vi "OpenSourceRIO.vi"() -> ()   [LabVIEW 2019]
uses:
  Controls/AnalogTrigger_Sources.ctl
  Controls/AnalogTrigger_Limits.ctl
  Controls/Encoder_Configs.ctl
  Controls/Encoder_Config.ctl
  Helpers/Source.ctl
  Controls/Encoder_TimerConfigs.ctl
  Controls/TimerConfig.ctl
  Controls/Interrupt_Configs.ctl
  Controls/DutyCycle_Sources.ctl
  Controls/Counter_TimerConfigs.ctl
  Controls/Counter_Configs.ctl
  Controls/Counter_Config.ctl
  Controls/Encoder_Output.ctl
  Helpers/TimerOutput.ctl
  Controls/Counter_Output.ctl
  Helpers/AnalogTriggerOutput.ctl
  <vilib>/Platform/TimedLoop/XDataNode/timing_clust.ctl
  <vilib>/Platform/TimedLoop/XDataNode/nitl_modes.ctl
  <vilib>/Platform/TimedLoop/XDataNode/wakeup.ctl
  <vilib>/rvi/Emulation/niFpgaGetClockAttributes.vi
  <vilib>/rvi/Emulation/niFpgaSctlEmulationGetInTimedLoop.vi
  <vilib>/rvi/Emulation/niFpgaEmulationReportErrorSimple.vi
  <vilib>/rvi/Emulation/niFpgaCriticalErrorInLSC.vi
  <vilib>/rvi/eio/common/nirviEmuTemplateMethod_errors.vi
  <vilib>/rvi/Emulation/niFpgaProcessEmulError.vi
  <vilib>/rvi/eio/common/nirviEmuTemplatePropertyGet_noerrors.vi
  <vilib>/rvi/occurrence/nirviWaitOnOccurrenceBase.vi
  <vilib>/eio/EIONode/EIONode.xnode
  <vilib>/eio/EIOPropertyNode/EIOPropertyNode.xnode
  <vilib>/platform/TimedLoop/XDataNode/XDataNode.xnode
  <vilib>/Platform/TimedLoop/XDataNode/XDNodeRunTimeDep.lvlib
  <vilib>/rvi/eio/common/nirviEmuTemplatePropertyGet_errors.vi
  <vilib>/rvi/eio/common/nirviEmuTemplatePropertySet_errors.vi
  <vilib>/rvi/eio/common/nirviEmuTemplatePropertySet_noerrors.vi
panel:
  in  "Relay3":u8
  in  "Relay2":u8
  in  "Relay1":u8
  in  "Relay0":u8
  in  "PWM_Squelch":u8[](array[numeric])=[0, 0, 0, 0, 0, 0, 0, 0, 0, 0]
  in  "PWM_0":u16=1500
  in  "PWM_2":u16
  in  "PWM_3":u16
  in  "PWM_4":u16
  in  "PWM_5":u16
  in  "PWM_6":u16
  in  "PWM_7":u16
  in  "PWM_8":u16
  in  "PWM_9":u16
  in  "PWM_1":u16
  in  "PWM_Period":u16=5005
  in  "PWM_MinHigh":u16=500
  out "Interrupt7_FallingTimestamp":u32
  out "Interrupt7_RisingTimestamp":u32
  out "Interrupt6_FallingTimestamp":u32
  out "Interrupt6_RisingTimestamp":u32
  out "Interrupt5_FallingTimestamp":u32
  out "Interrupt5_RisingTimestamp":u32
  out "Interrupt4_FallingTimestamp":u32
  out "Interrupt4_RisingTimestamp":u32
  out "Interrupt3_FallingTimestamp":u32
  out "Interrupt3_RisingTimestamp":u32
  out "Interrupt2_FallingTimestamp":u32
  out "Interrupt2_RisingTimestamp":u32
  out "Interrupt1_FallingTimestamp":u32
  out "Interrupt1_RisingTimestamp":u32
  out "Interrupt0_FallingTimestamp":u32
  out "Interrupt0_RisingTimestamp":u32
  out "AT7_Output":T1
  out "AT6_Output":T1
  out "AT5_Output":T1
  out "AT4_Output":T1
  out "AT3_Output":T1
  out "AT2_Output":T1
  out "AT1_Output":T1
  out "AT0_Output":T1
  out "Counter7_TimerOutput":T2
  out "Counter6_TimerOutput":T2
  out "Counter5_TimerOutput":T2
  out "Counter4_TimerOutput":T2
  out "Counter3_TimerOutput":T2
  out "Counter2_TimerOutput":T2
  out "Counter1_TimerOutput":T2
  out "Counter0_TimerOutput":T2
  out "Counter7_Output":T3
  out "Counter6_Output":T3
  out "Counter5_Output":T3
  out "Counter4_Output":T3
  out "Counter3_Output":T3
  out "Counter2_Output":T3
  out "Counter1_Output":T3
  out "Counter0_Output":T3
  out "Encoder7_TimerOutput":T2
  out "Encoder6_TimerOutput":T2
  out "Encoder5_TimerOutput":T2
  out "Encoder4_TimerOutput":T2
  out "Encoder3_TimerOutput":T2
  out "Encoder2_TimerOutput":T2
  out "Encoder1_TimerOutput":T2
  out "Encoder0_TimerOutput":T2
  out "Encoder7_Output":T4
  out "Encoder6_Output":T4
  out "Encoder5_Output":T4
  out "Encoder4_Output":T4
  out "Encoder3_Output":T4
  out "Encoder2_Output":T4
  out "Encoder1_Output":T4
  out "Encoder0_Output":T4
  in  "Counter7_Reset":bool
  in  "Counter6_Reset":bool
  in  "Counter5_Reset":bool
  in  "Counter4_Reset":bool
  in  "Counter3_Reset":bool
  in  "Counter2_Reset":bool
  in  "Counter1_Reset":bool
  in  "Counter0_Reset":bool
  in  "Encoder7_Reset":bool
  in  "Encoder6_Reset":bool
  in  "Encoder5_Reset":bool
  in  "Encoder4_Reset":bool
  in  "Encoder3_Reset":bool
  in  "Encoder2_Reset":bool
  in  "Encoder1_Reset":bool
  in  "Encoder0_Reset":bool
  out "DutyCycle7_Output":fxp<+,31,31>
  out "DutyCycle6_Output":fxp<+,31,31>
  out "DutyCycle5_Output":fxp<+,31,31>
  out "DutyCycle4_Output":fxp<+,31,31>
  out "DutyCycle3_Output":fxp<+,31,31>
  out "DutyCycle2_Output":fxp<+,31,31>
  out "DutyCycle1_Output":fxp<+,31,31>
  out "DutyCycle0_Output":fxp<+,31,31>
  out "DutyCycle7_Frequency":fxp<+,11,11>
  out "DutyCycle6_Frequency":fxp<+,11,11>
  out "DutyCycle5_Frequency":fxp<+,11,11>
  out "DutyCycle4_Frequency":fxp<+,11,11>
  out "DutyCycle3_Frequency":fxp<+,11,11>
  out "DutyCycle2_Frequency":fxp<+,11,11>
  out "DutyCycle1_Frequency":fxp<+,11,11>
  out "DutyCycle0_Frequency":fxp<+,11,11>
  in  "Counter_Configs":T5
  in  "Counter_TimerConfigs":T8
  in  "DutyCycle_Sources":T10
  in  "Interrupts_Configs":T11
  in  "Encoder_TimerConfigs":T12
  in  "Encoder_Configs":T13
  in  "AnalogTrigger_Limits":T15
  in  "AnalogTrigger_Sources":T16
  in  "SPI_DIOEnable":u8
  in  "Digital_Outputs":u32
  in  "Digital_Output_Directions":u32
  in  "InterruptForceNumber":u8
  in  "InterruptForceOnce":bool
  in  "PWM_FeedWatchdog":bool
  out "AnalogInputs":u16[](array[numeric])
  in  "Analog_SampleRate":u32=100
  out "AccelerationX":i16
  out "AccelerationY":i16
  out "AccelerationZ":i16
  out "Analog_Offset":i32
  out "Analog_LSBWeight":u32
  in  "Analog_AO1":u16
  in  "Analog_AO0":u16
  out "Analog_AI7":u16
  out "Analog_AI6":u16
  out "Analog_AI5":u16
  out "Analog_AI4":u16
  out "Analog_AI3":u16
  out "Analog_AI2":u16
  out "Analog_AI1":u16
  out "Analog_AI0":u16
  in  "Alarm_TriggerTime":u32
  in  "Alarm_Enable":bool
  out "Digital_Inputs":u32
  in  "Mode_LED_Red":bool
  in  "Comm_LED_Red":bool
  in  "Mode_LED_Green":bool
  in  "Comm_LED_Green":bool
  in  "Radio_LED_Red":bool
  in  "Radio_LED_Green":bool
  out "User_Button":bool
  out "Timing_Upper":u32
  out "Timing_Lower":u32
  in  "Timing_Reset":bool
  out "Num_Digital_Inputs":u8
  out "PWM_Enabled":bool
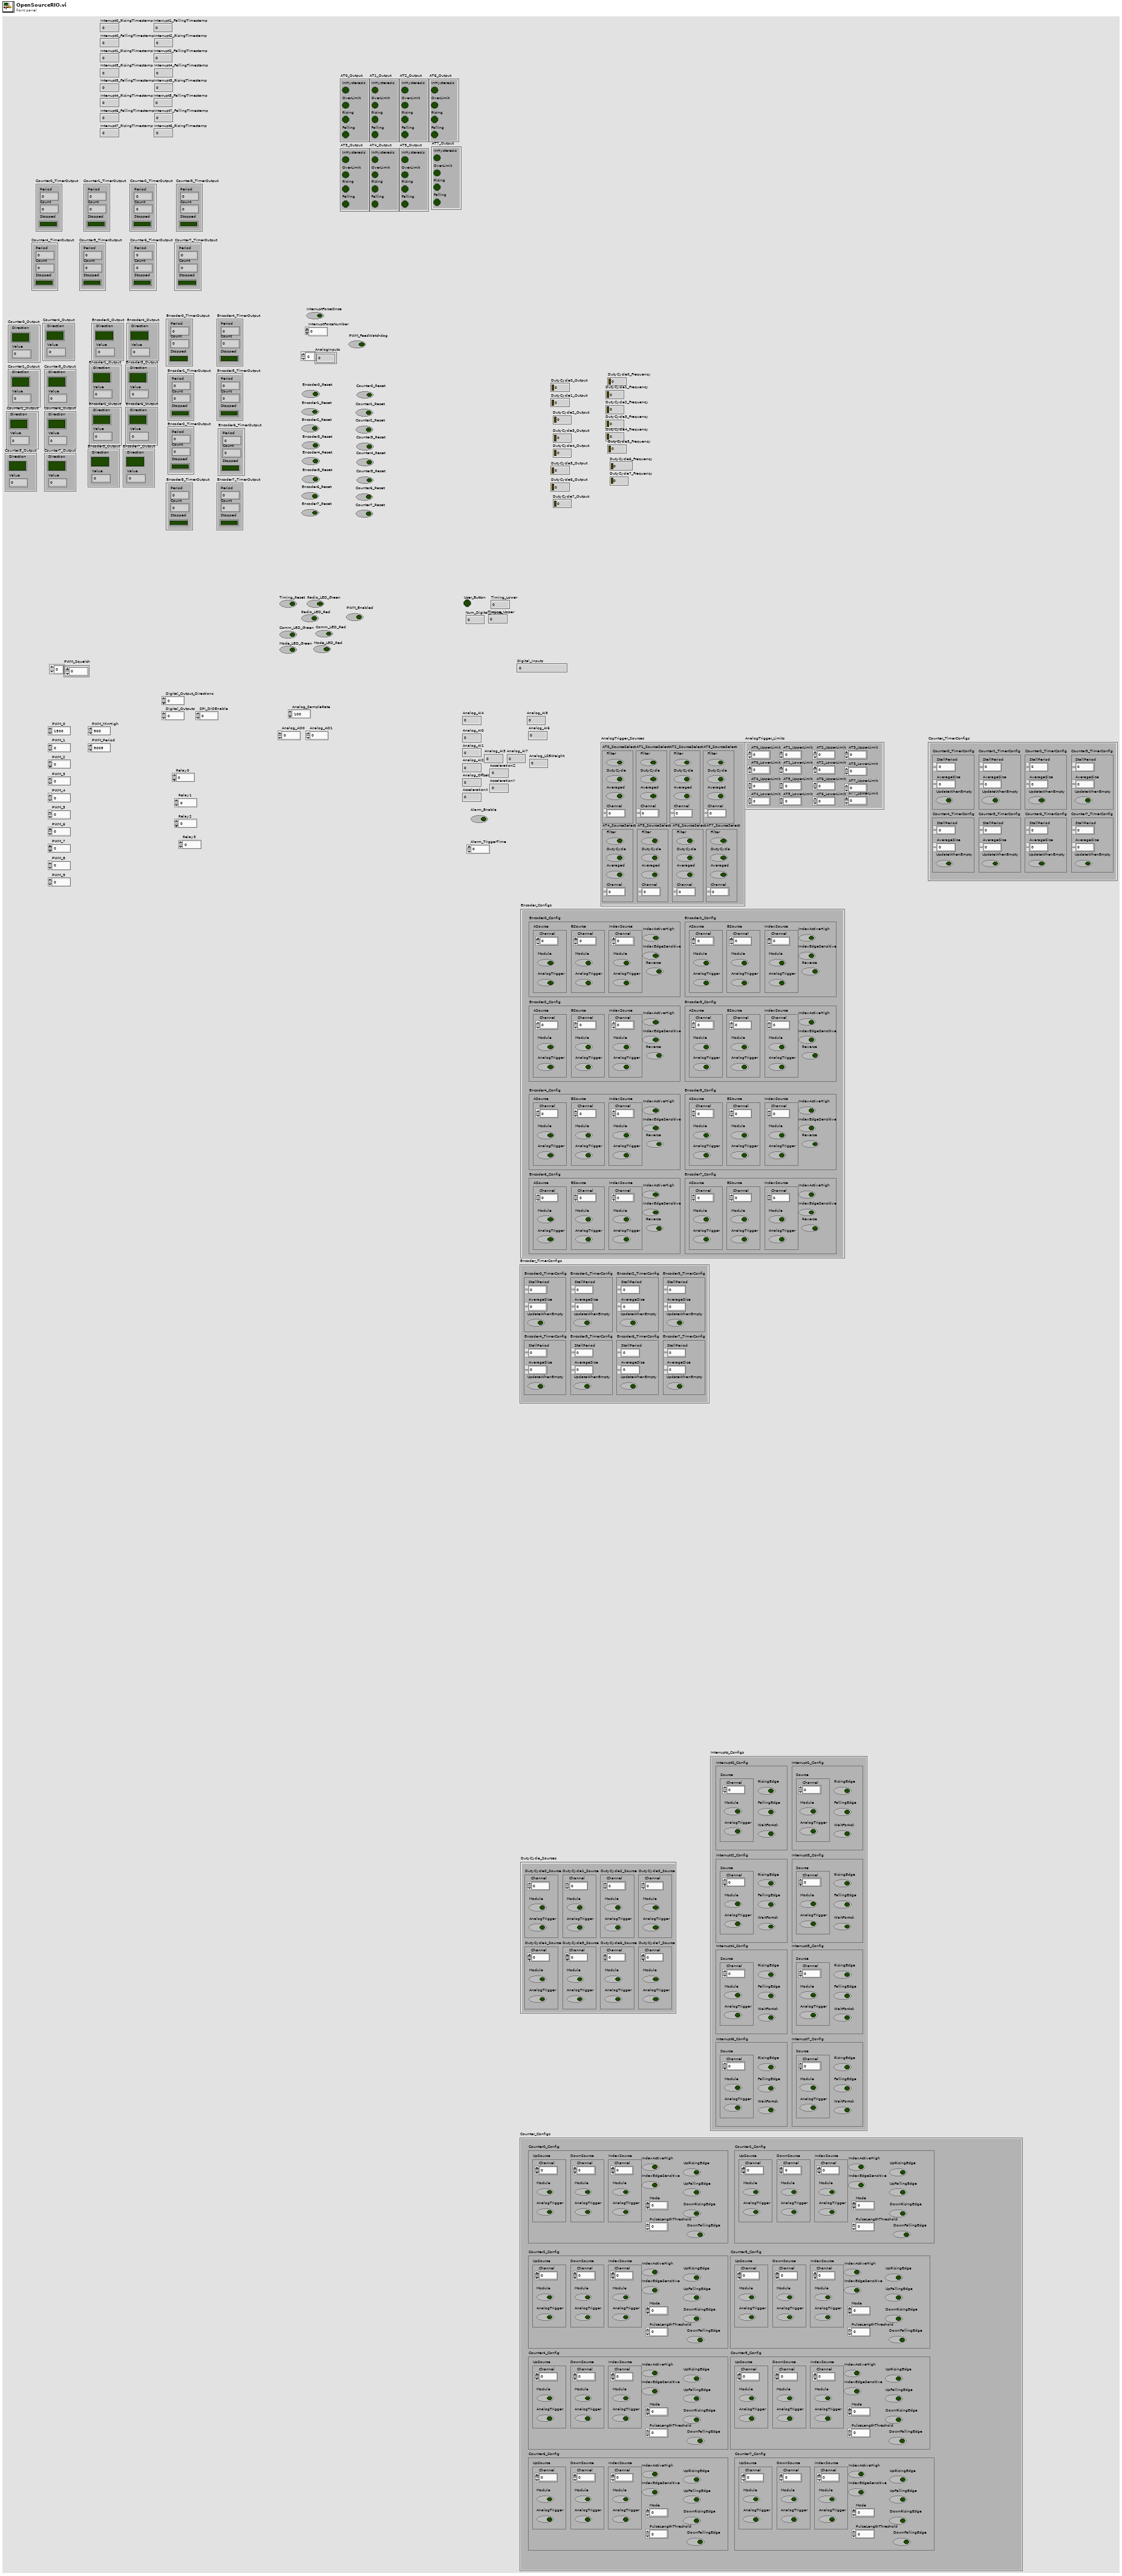
[diagram p1: front panel]
types:
  T1 = typedef "AnalogTriggerOutput.ctl" = cluster{"InHysteresis":bool, "OverLimit":bool, "Rising":bool, "Falling":bool}
  T2 = typedef "TimerOutput.ctl" = cluster{"Period":fxp<+,24,25>, "Count":i16, "Stopped":bool}
  T3 = typedef "Counter_Output.ctl" = cluster{"Direction":bool, "Value":fxp<+/-,31,31>}
  T4 = typedef "Encoder_Output.ctl" = cluster{"Direction":bool, "Value":fxp<+/-,31,31>}
  T5 = typedef "Counter_Configs.ctl" = cluster{"Counter0_Config":T6, "Counter1_Config":T6, "Counter2_Config":T6, "Counter3_Config":T6, "Counter4_Config":T6, "Counter5_Config":T6, "Counter6_Config":T6, "Counter7_Config":T6}
  T6 = typedef "Counter_Config.ctl" = cluster{"UpSource":T7, "DownSource":T7, "IndexSource":T7, "IndexActiveHigh":bool, "IndexEdgeSensitive":bool, "UpRisingEdge":bool, "UpFallingEdge":bool, "DownRisingEdge":bool, "DownFallingEdge":bool, "Mode":fxp<+,2,2>, "PulseLengthThreshold":fxp<+,6,14>}
  T7 = typedef "Source.ctl" = cluster{"Channel":fxp<+,4,4>, "Module":bool, "AnalogTrigger":bool}
  T8 = typedef "Counter_TimerConfigs.ctl" = cluster{"Counter0_TimerConfig":T9, "Counter1_TimerConfig":T9, "Counter2_TimerConfig":T9, "Counter3_TimerConfig":T9, "Counter4_TimerConfig":T9, "Counter5_TimerConfig":T9, "Counter6_TimerConfig":T9, "Counter7_TimerConfig":T9}
  T9 = typedef "TimerConfig.ctl" = cluster{"StallPeriod":fxp<+,24,24>, "AverageSize":fxp<+,7,7>, "UpdateWhenEmpty":bool}
  T10 = typedef "DutyCycle_Sources.ctl" = cluster{"DutyCycle0_Source":T7, "DutyCycle1_Source":T7, "DutyCycle2_Source":T7, "DutyCycle3_Source":T7, "DutyCycle4_Source":T7, "DutyCycle5_Source":T7, "DutyCycle6_Source":T7, "DutyCycle7_Source":T7}
  T11 = typedef "Interrupt_Configs.ctl" = cluster{"Interrupt0_Config":cluster{"Source":T7, "RisingEdge":bool, "FallingEdge":bool, "WaitForAck":bool}, "Interrupt1_Config":cluster{"Source":T7, "RisingEdge":bool, "FallingEdge":bool, "WaitForAck":bool}, "Interrupt2_Config":cluster{"Source":T7, "RisingEdge":bool, "FallingEdge":bool, "WaitForAck":bool}, "Interrupt3_Config":cluster{"Source":T7, "RisingEdge":bool, "FallingEdge":bool, "WaitForAck":bool}, "Interrupt4_Config":cluster{"Source":T7, "RisingEdge":bool, "FallingEdge":bool, "WaitForAck":bool}, "Interrupt5_Config":cluster{"Source":T7, "RisingEdge":bool, "FallingEdge":bool, "WaitForAck":bool}, "Interrupt6_Config":cluster{"Source":T7, "RisingEdge":bool, "FallingEdge":bool, "WaitForAck":bool}, "Interrupt7_Config":cluster{"Source":T7, "RisingEdge":bool, "FallingEdge":bool, "WaitForAck":bool}}
  T12 = typedef "Encoder_TimerConfigs.ctl" = cluster{"Encoder0_TimerConfig":T9, "Encoder1_TimerConfig":T9, "Encoder2_TimerConfig":T9, "Encoder3_TimerConfig":T9, "Encoder4_TimerConfig":T9, "Encoder5_TimerConfig":T9, "Encoder6_TimerConfig":T9, "Encoder7_TimerConfig":T9}
  T13 = typedef "Encoder_Configs.ctl" = cluster{"Encoder0_Config":T14, "Encoder1_Config":T14, "Encoder2_Config":T14, "Encoder3_Config":T14, "Encoder4_Config":T14, "Encoder5_Config":T14, "Encoder6_Config":T14, "Encoder7_Config":T14}
  T14 = typedef "Encoder_Config.ctl" = cluster{"ASource":T7, "BSource":T7, "IndexSource":T7, "IndexActiveHigh":bool, "IndexEdgeSensitive":bool, "Reverse":bool}
  T15 = typedef "AnalogTrigger_Limits.ctl" = cluster{"AT0_LowerLimit":u32, "AT0_UpperLimit":u32, "AT1_LowerLimit":u32, "AT1_UpperLimit":u32, "AT2_LowerLimit":u32, "AT2_UpperLimit":u32, "AT3_LowerLimit":u32, "AT3_UpperLimit":u32, "AT4_LowerLimit":u32, "AT4_UpperLimit":u32, "AT5_LowerLimit":u32, "AT5_UpperLimit":u32, "AT6_LowerLimit":u32, "AT6_UpperLimit":u32, "AT7_LowerLimit":u32, "AT7_UpperLimit":u32}
  T16 = typedef "AnalogTrigger_Sources.ctl" = cluster{"AT0_SourceSelect":cluster{"Filter":bool, "DutyCycle":bool, "Averaged":bool, "Channel":fxp<+,3,3>}, "AT1_SourceSelect":cluster{"Filter":bool, "DutyCycle":bool, "Averaged":bool, "Channel":fxp<+,3,3>}, "AT2_SourceSelect":cluster{"Filter":bool, "DutyCycle":bool, "Averaged":bool, "Channel":fxp<+,3,3>}, "AT3_SourceSelect":cluster{"Filter":bool, "DutyCycle":bool, "Averaged":bool, "Channel":fxp<+,3,3>}, "AT4_SourceSelect":cluster{"Filter":bool, "DutyCycle":bool, "Averaged":bool, "Channel":fxp<+,3,3>}, "AT5_SourceSelect":cluster{"Filter":bool, "DutyCycle":bool, "Averaged":bool, "Channel":fxp<+,3,3>}, "AT6_SourceSelect":cluster{"Filter":bool, "DutyCycle":bool, "Averaged":bool, "Channel":fxp<+,3,3>}, "AT7_SourceSelect":cluster{"Filter":bool, "DutyCycle":bool, "Averaged":bool, "Channel":fxp<+,3,3>}}
  T17 = typedef "XDNodeRunTimeDep.lvlib/timing_clust.ctl" = cluster{"Expected End [f-1]":u64, "Actual End [f-1]":u64, "Finished Late? [f-1]":bool, "Expected End [i-1]":u64, "Actual End [i-1]":u64, "Finished Late? [i-1]":bool, "Expected Start [i]":u64, "Actual Start [i]":u64, "Expected Start [f]":u64, "Actual Start [f]":u64, "Source Name":string, "Structure Name":string, "Period":i64, "Deadline":i64, "Offset":i64, "Start":i64, "Priority":i32, "Timeout":i32, "Mode":T18, "Wakeup Reason":T19, "Error":errorcluster, "Source Type":string, "Secondary Source Type":string, "Global End Time":u64, "Global Start Time":u64, "Frame Duration":u64, "Iteration Duration":u64, "Assigned CPU":i32, "I/O Scan Engine Mode":u32}
  T18 = typedef "XDNodeRunTimeDep.lvlib/nitl_modes.ctl" = enum32{"No Change", "Process missed periods, maintain original phase", "Discard missed periods, maintain original phase", "Process missed periods, ignore original phase", "Discard missed periods, ignore original phase"}
  T19 = typedef "XDNodeRunTimeDep.lvlib/wakeup.ctl" = enum32{"Normal", "Aborted", "Asynchronous wakeup", "Timing source error", "Timed loop error", "Timeout"}
  T20 = cluster{"[0]":bool, "[1]":bool, "[2]":bool, "[3]":bool, "[4]":bool, "[5]":bool, "[6]":bool, "[7]":bool, "[8]":bool, "[9]":bool}
  T21 = cluster{"Boolean array[0]":bool, "Boolean array[1]":bool}
  T22 = typedef "Interrupt_Occurances.ctl" = cluster{"Interrupt0_Rising":refnum<k4>, "Interrupt0_Falling":refnum<k4>, "Interrupt1_Rising":refnum<k4>, "Interrupt1_Falling":refnum<k4>, "Interrupt2_Rising":refnum<k4>, "Interrupt2_Falling":refnum<k4>, "Interrupt3_Rising":refnum<k4>, "Interrupt3_Falling":refnum<k4>, "Interrupt4_Rising":refnum<k4>, "Interrupt4_Falling":refnum<k4>, "Interrupt5_Rising":refnum<k4>, "Interrupt5_Falling":refnum<k4>, "Interrupt6_Rising":refnum<k4>, "Interrupt6_Falling":refnum<k4>, "Interrupt7_Rising":refnum<k4>, "Interrupt7_Falling":refnum<k4>}
  T23 = typedef "DutyCycle_Frequencies.ctl" = cluster{"DutyCycle0_Frequency":fxp<+,11,11>, "DutyCycle1_Frequency":fxp<+,11,11>, "DutyCycle2_Frequency":fxp<+,11,11>, "DutyCycle3_Frequency":fxp<+,11,11>, "DutyCycle4_Frequency":fxp<+,11,11>, "DutyCycle5_Frequency":fxp<+,11,11>, "DutyCycle6_Frequency":fxp<+,11,11>, "DutyCycle7_Frequency":fxp<+,11,11>}
  T24 = typedef "DutyCycle_Outputs.ctl" = cluster{"DutyCycle0_Output":fxp<+,31,31>, "DutyCycle1_Output":fxp<+,31,31>, "DutyCycle2_Output":fxp<+,31,31>, "DutyCycle3_Output":fxp<+,31,31>, "DutyCycle4_Output":fxp<+,31,31>, "DutyCycle5_Output":fxp<+,31,31>, "DutyCycle6_Output":fxp<+,31,31>, "DutyCycle7_Output":fxp<+,31,31>}
  T25 = typedef "AnalogTrigger_Outputs.ctl" = cluster{"AT0_Output":T1, "AT1_Output":T1, "AT2_Output":T1, "AT3_Output":T1, "AT4_Output":T1, "AT5_Output":T1, "AT6_Output":T1, "AT7_Output":T1}
  T26 = cluster{"Counter0_Reset":bool, "Counter1_Reset":bool, "Counter2_Reset":bool, "Counter3_Reset":bool, "Counter4_Reset":bool, "Counter5_Reset":bool, "Counter6_Reset":bool, "Counter7_Reset":bool}
  T27 = typedef "Interrupt_Timestamps.ctl" = cluster{"Interrupt0_RisingTimestamp":u32, "Interrupt0_FallingTimestamp":u32, "Interrupt1_RisingTimestamp":u32, "Interrupt1_FallingTimestamp":u32, "Interrupt2_RisingTimestamp":u32, "Interrupt2_FallingTimestamp":u32, "Interrupt3_RisingTimestamp":u32, "Interrupt3_FallingTimestamp":u32, "Interrupt4_RisingTimestamp":u32, "Interrupt4_FallingTimestamp":u32, "Interrupt5_RisingTimestamp":u32, "Interrupt5_FallingTimestamp":u32, "Interrupt6_RisingTimestamp":u32, "Interrupt6_FallingTimestamp":u32, "Interrupt7_RisingTimestamp":u32, "Interrupt7_FallingTimestamp":u32}
  T28 = typedef "Counter_Outputs.ctl" = cluster{"Counter0_Output":T3, "Counter1_Output":T3, "Counter2_Output":T3, "Counter3_Output":T3, "Counter4_Output":T3, "Counter5_Output":T3, "Counter6_Output":T3, "Counter7_Output":T3}
  T29 = typedef "Counter_TimerOutputs.ctl" = cluster{"Counter0_TimerOutput":T2, "Counter1_TimerOutput":T2, "Counter2_TimerOutput":T2, "Counter3_TimerOutput":T2, "Counter4_TimerOutput":T2, "Counter5_TimerOutput":T2, "Counter6_TimerOutput":T2, "Counter7_TimerOutput":T2}
  T30 = cluster{"Encoder0_Reset":bool, "Encoder1_Reset":bool, "Encoder2_Reset":bool, "Encoder3_Reset":bool, "Encoder4_Reset":bool, "Encoder5_Reset":bool, "Encoder6_Reset":bool, "Encoder7_Reset":bool}
  T31 = typedef "Encoder_Outputs.ctl" = cluster{"Encoder0_Output":T4, "Encoder1_Output":T4, "Encoder2_Output":T4, "Encoder3_Output":T4, "Encoder4_Output":T4, "Encoder5_Output":T4, "Encoder6_Output":T4, "Encoder7_Output":T4}
  T32 = typedef "Encoder_TimerOutputs.ctl" = cluster{"Encoder0_TimerOutput":T2, "Encoder1_TimerOutput":T2, "Encoder2_TimerOutput":T2, "Encoder3_TimerOutput":T2, "Encoder4_TimerOutput":T2, "Encoder5_TimerOutput":T2, "Encoder6_TimerOutput":T2, "Encoder7_TimerOutput":T2}
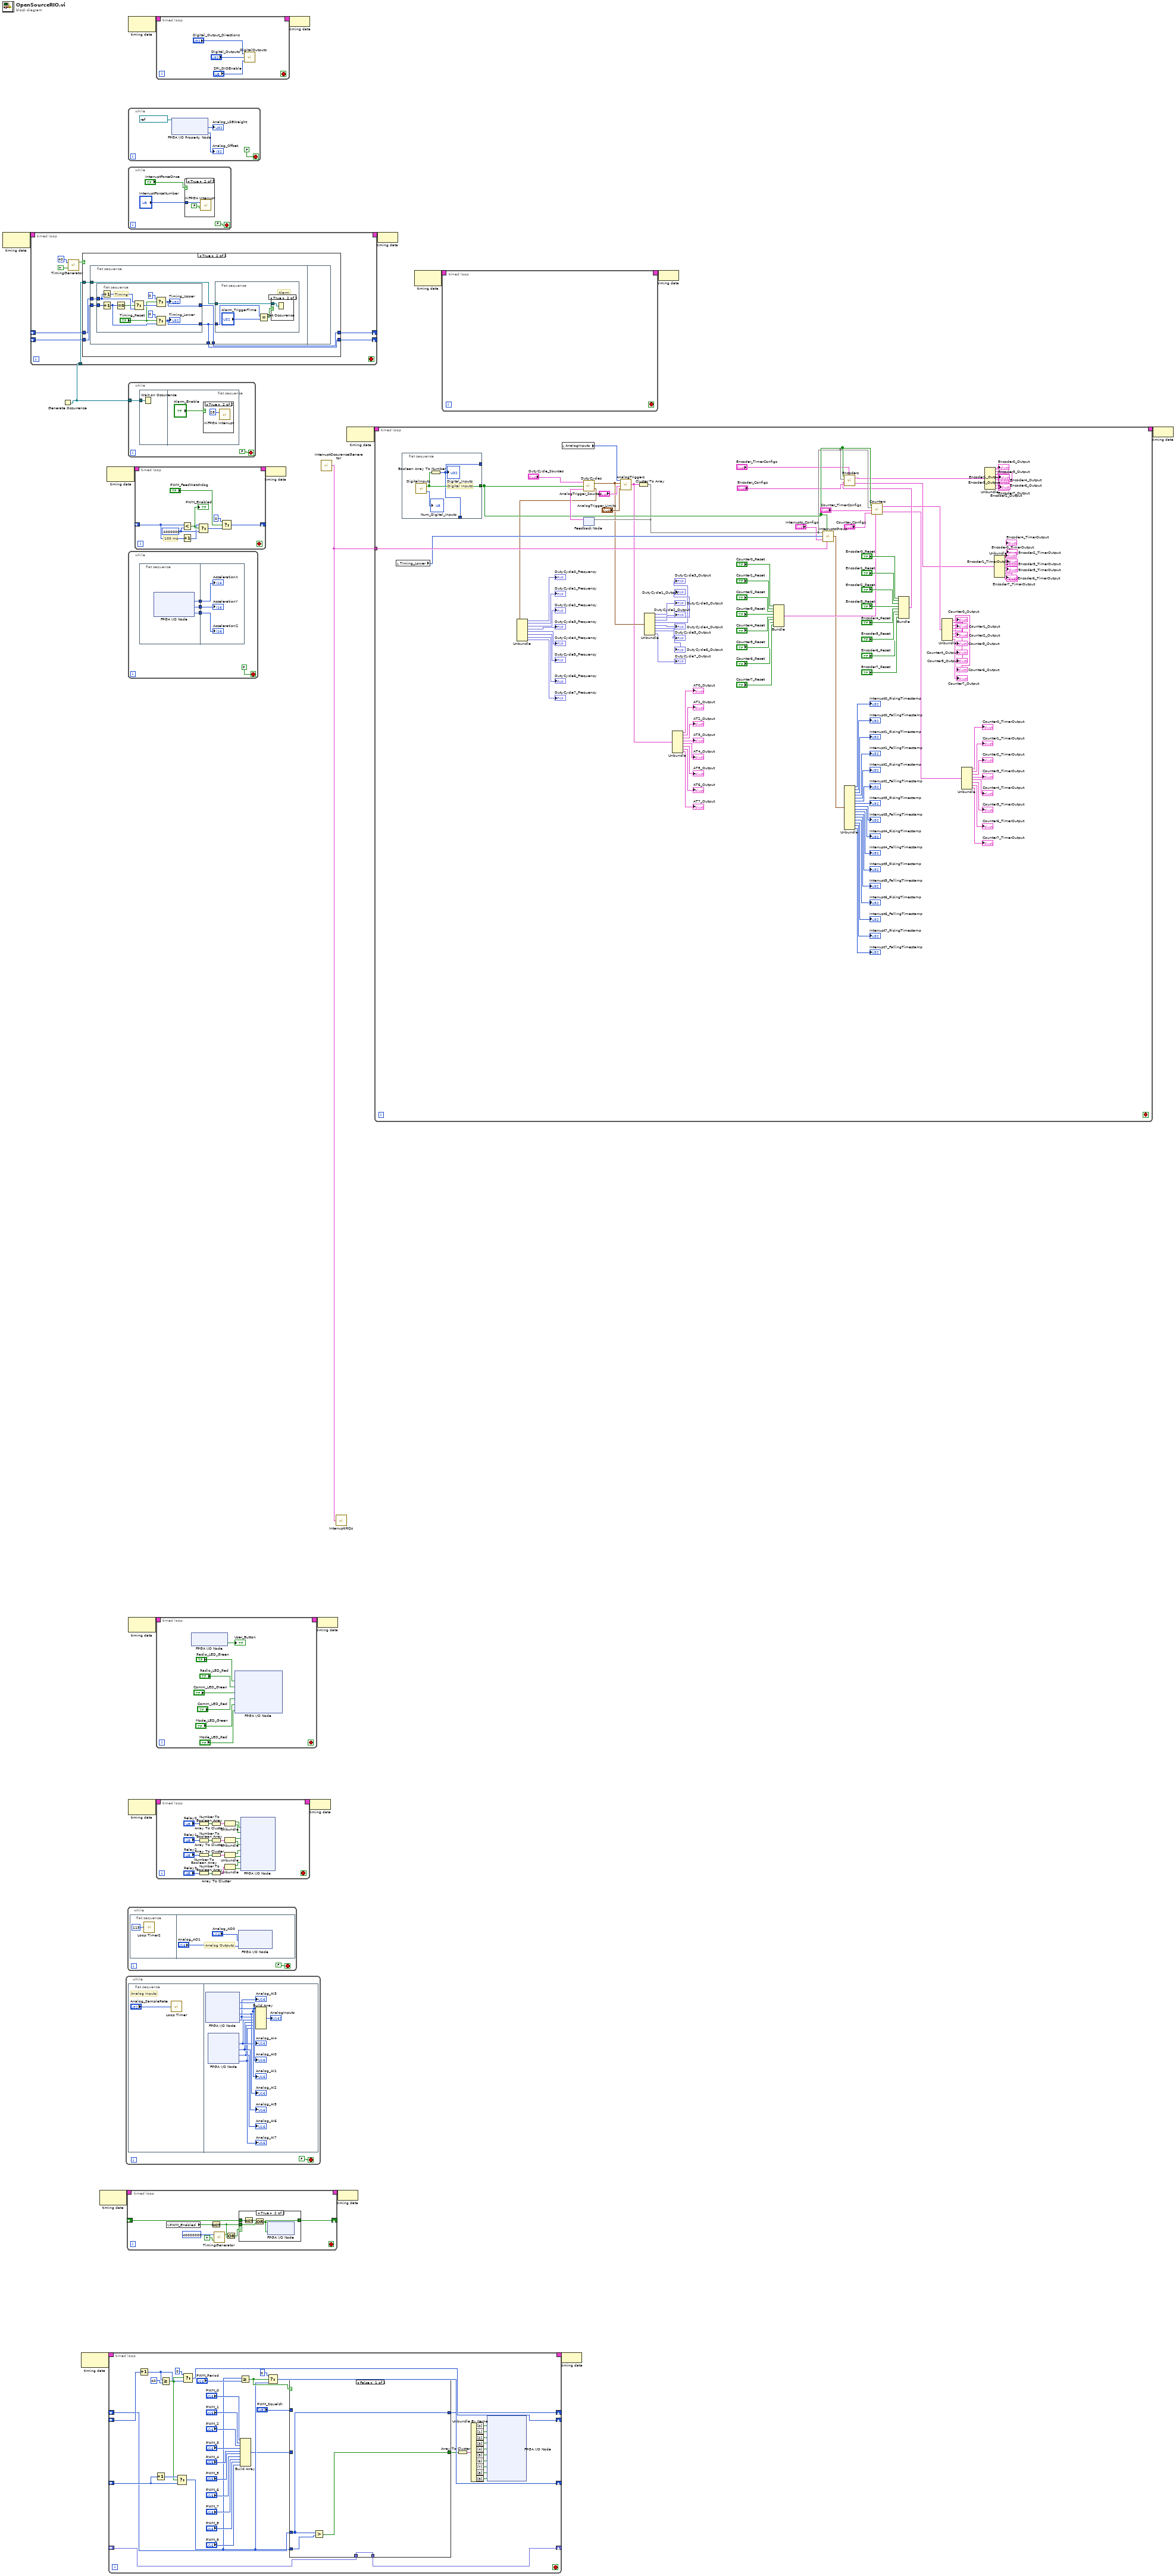
[diagram p0: block diagram]
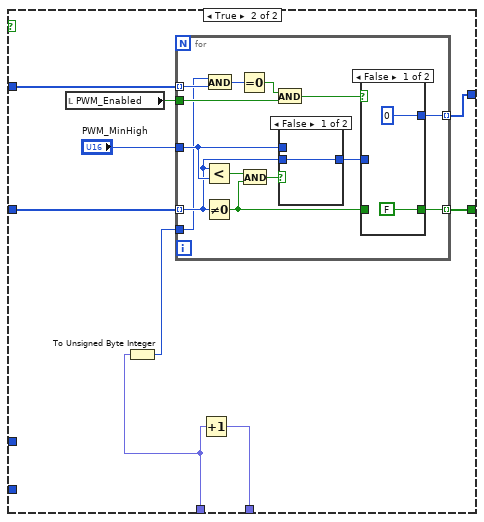
[diagram p2: hidden frame]
diagram:
  n1 = node-c288() -> (w20:T17)  [unwired: 1 in]
  n2 = Generate Occurrence() -> (w8:refnum<k4>)
  n3 = timed-loop {
    timing: w20 -> [_]
    timing-out: [_] -> w19
    shift-right: [w25] -> _
    shift-left: _ -> [w23]
    shift-right: [w24] -> _
    shift-left: _ -> [w22]
    tunnel: w8 -> [w21]
    stop <- _ stop-if-true
    n4 = call "TimingGenerator.vi"("Tick"=TRUE, "Period"=u32 40) -> ("Pulse"=w26:bool)  [unwired: 1 out]
    n5 = case shown="True" w26 {
      tunnel: [w29 w35] -> w25
      tunnel: [w30 w34] -> w24
      tunnel: w23 -> [w29 w33]
      tunnel: w22 -> [w30 w32]
      tunnel: w21 -> [_ w31]
      frame False {
      }
      frame True {
        n6 = flat-sequence {
          tunnel: [w40] -> w35
          tunnel: [w37] -> w34
          tunnel: w33 -> [w39]
          tunnel: w32 -> [w38]
          tunnel: w31 -> [w36]
          frame #0 {
            n7 = flat-sequence {
              tunnel: [w46] -> w40
              tunnel: w39 -> [w45]
              tunnel: w38 -> [w44]
              tunnel: [w41] -> w37
              frame #0 {
                # "Timing"
                n8 = Increment(x=w45) -> (x+1=w50:u32)
                n9 = Increment(x=w44) -> (x+1=w43:u32)
                n10 = Equal To 0?(x=w43) -> (x = 0?=w42:bool)
                n11 = Select(t=w50, s=w42, f=w45) -> (s? t:f=w51:u32)
                n12 = Select(t=u32 0, s="Timing_Reset", f=w51) -> (s? t:f=w46:u32)
                "Timing_Upper" <- w46
                n13 = Select(t=u32 0, s="Timing_Reset", f=w43) -> (s? t:f=w41:u32)
                "Timing_Lower" <- w41
              }
            }
            n14 = flat-sequence {
              tunnel: w37 -> [w53]
              tunnel: w36 -> [w52]
              frame #0 {
                # "Alarm"
                n15 = Equal?(x=w53, y="Alarm_TriggerTime") -> (x = y?=w55:bool)
                n16 = case shown="True" w55 {
                  tunnel: w52 -> [_ w56]
                  frame False {
                  }
                  frame True {
                    n17 = Set Occurrence(w56) -> ()
                  }
                }
              }
            }
          }
          frame #1 {
          }
        }
      }
    }
  }
  n18 = node-c288() -> (w2:T17)  [unwired: 1 in]
  n19 = node-c288() -> (w18:T17)  [unwired: 1 in]
  n20 = node-c288() -> (w12:T17)  [unwired: 1 in]
  n21 = timed-loop {
    timing: w2 -> [_]
    timing-out: [_] -> w1
    shift-right: [w76] -> _
    shift-left: _ -> [w79]
    shift-right: [w98] -> _
    shift-left: _ -> [w97]
    shift-right: [w86] -> _
    shift-left: _ -> [w83]
    shift-right: [w59] -> _
    shift-left: _ -> [w60]
    stop <- _ stop-if-true
    n22 = Increment(x=w97) -> (x+1=w61:u8)
    n23 = Increment(x=w83) -> (x+1=w84:u16)
    n24 = Greater Or Equal?(x=w61, y=u8 40 ("x")) -> (x >= y?=w81:bool)
    n25 = Select(t=w84, s=w81, f=w83) -> (s? t:f=w78:u16)
    n26 = Select(t=u8 0, s=w81, f=w61) -> (s? t:f=w98:u8)
    n27 = Greater Or Equal?(x=w78, y="PWM_Period") -> (x >= y?=w80:bool)
    n28 = Build Array("PWM_0", "PWM_1", "PWM_2", "PWM_3", "PWM_4", "PWM_5", "PWM_6", "PWM_7", "PWM_8", "PWM_9") -> (w77:u16[])
    n29 = Select(t=u16 0, s=w80, f=w78) -> (s? t:f=w86:u16)
    n30 = case shown="False" w80 {
      tunnel: w79 -> [w101 _]
      tunnel: w78 -> [w103 _]
      tunnel: [w102 w109] -> w64
      tunnel: w77 -> [_ w112]
      tunnel: [w101 w111] -> w76
      tunnel: "PWM_Squelch" -> [_ w107]
      tunnel: w60 -> [w100 w105]
      tunnel: [w100 w106] -> w59
      frame False {
        n31 = Greater?(x=w101, y=w103) -> (0:w102:bool[])
      }
      frame True {
        n32 = local read "PWM_Enabled"() -> (w108:bool)
        n33 = To Unsigned Byte Integer(number=w105) -> (unsigned 8bit integer=w104:u8)
        n34 = for {
          tunnel: w112 -> [w123] mode=indexing
          tunnel: [w121] -> w111 mode=indexing
          tunnel: [w119] -> w109 mode=indexing
          tunnel: "PWM_MinHigh" -> [w124]
          tunnel: w108 -> [w116]
          tunnel: w107 -> [w120] mode=indexing
          tunnel: w104 -> [w113]
          n35 = Less?(x=w123, y=w124) -> (x < y?=w126:bool)
          n36 = Not Equal To 0?(x=w123) -> (x != 0?=w114:bool)
          n37 = And(x=w113, y=w120) -> (x .and. y?=w118:u8)
          n38 = Equal To 0?(x=w118) -> (x = 0?=w117:bool)
          n39 = And(x=w126, y=w114) -> (x .and. y?=w125:bool)
          n40 = And(x=w117, y=w116) -> (x .and. y?=w115:bool)
          n41 = case shown="False" w125 {
            tunnel: [w131 w132] -> w122
            tunnel: w124 -> [_ w132]
            tunnel: w123 -> [w131 _]
            frame False {
            }
            frame True {
            }
          }
          n42 = case shown="False" w115 {
            tunnel: [u16 0 ("PWM_MinHigh") w130] -> w121
            tunnel: w122 -> [_ w130]
            tunnel: [FALSE w129] -> w119
            tunnel: w114 -> [_ w129]
            frame False {
            }
            frame True {
            }
          }
        }
        n43 = Increment(x=w105) -> (x+1=w106:fxp<+,2,2>)
      }
    }
    n44 = Array To Cluster(array=w64) -> (cluster=w75:T20)
    n45 = Unbundle By Name(w75) -> ("[0]"=w74:bool, "[1]"=w73:bool, "[2]"=w72:bool, "[3]"=w71:bool, "[4]"=w70:bool, "[5]"=w69:bool, "[6]"=w68:bool, "[7]"=w67:bool, "[8]"=w66:bool, "[9]"=w65:bool)
    n46 = xnode "FPGA I/O Node"("PWM/PWM0"=w74, "PWM/PWM1"=w73, "PWM/PWM2"=w72, "PWM/PWM3"=w71, "PWM/PWM4"=w70, "PWM/PWM5"=w69, "PWM/PWM6"=w68, "PWM/PWM7"=w67, "PWM/PWM8"=w66, "PWM/PWM9"=w65) -> ()  [unwired: 10 in, 10 out]
  }
  n47 = while {
    stop <- FALSE stop-if-true
    n48 = flat-sequence {
      frame #0 {
        # "Analog Inputs"
        n49 = call "Loop Timer"("Count(Ticks)"="Analog_SampleRate") -> ()  [unwired: 1 out]
      }
      frame #1 {
        n50 = xnode "FPGA I/O Node"() -> ("AnalogIn0"=w145:u16, "AnalogIn1"=w144:u16, "AnalogIn2"=w143:u16, "AnalogIn3"=w142:u16)  [unwired: 4 in, 4 out]
        "Analog_AI0" <- w145
        "Analog_AI1" <- w144
        "Analog_AI2" <- w143
        "Analog_AI3" <- w142
        n51 = xnode "FPGA I/O Node"() -> ("MXP/AI0"=w141:u16, "MXP/AI1"=w140:u16, "MXP/AI2"=w139:u16, "MXP/AI3"=w138:u16)  [unwired: 4 in, 4 out]
        "Analog_AI4" <- w141
        "Analog_AI5" <- w140
        "Analog_AI6" <- w139
        "Analog_AI7" <- w138
        n52 = Build Array(w145, w144, w143, w142, w141, w140, w139, w138) -> (→"AnalogInputs":u16[])
      }
    }
  }
  n53 = timed-loop {
    timing: w18 -> [_]
    timing-out: [_] -> w17
    shift-right: [w147] -> _
    shift-left: _ -> [w146]
    stop <- _ stop-if-true
    n54 = local read "PWM_Enabled"() -> (w150:bool)
    n55 = Not(x=w150) -> (.not. x?=w148:bool)
    n56 = call "TimingGenerator.vi"("Tick"=TRUE, "Period"=u32 40000000) -> ("Pulse"=w151:bool)  [unwired: 1 out]
    n57 = Or(x=w151, y=w148) -> (x .or. y?=w149:bool)
    n58 = case shown="True" w149 {
      tunnel: w146 -> [w154 w158]
      tunnel: w148 -> [_ w156]
      tunnel: [w154 w155] -> w147
      frame False {
      }
      frame True {
        n59 = Not(x=w158) -> (.not. x?=w157:bool)
        n60 = Or(x=w157, y=w156) -> (x .or. y?=w155:bool)
        n61 = xnode "FPGA I/O Node"("RSL"=w155) -> ()  [unwired: 1 in, 1 out]
      }
    }
  }
  n62 = while {
    stop <- FALSE stop-if-true
    n63 = flat-sequence {
      frame #0 {
        n64 = call "Loop Timer2"("Count(Ticks)"=u32 115) -> ()  [unwired: 1 out]
      }
      frame #1 {
        # "Analog Outputs"
        n65 = xnode "FPGA I/O Node"("MXP/AO0"="Analog_AO0", "MXP/AO1"="Analog_AO1") -> ()  [unwired: 2 in, 2 out]
      }
    }
  }
  n66 = node-c288() -> (w10:T17)  [unwired: 1 in]
  n67 = while {
    stop <- FALSE stop-if-true
    n68 = xnode "FPGA I/O Property Node"("FPGA I/O In"=refnum<k21> "AnalogIn0") -> ("LSB Weight"=→"Analog_LSBWeight":u32, "Offset"=→"Analog_Offset":i32)  [unwired: 1 out]
  }
  n69 = while {
    stop <- FALSE stop-if-true
    n70 = case shown="True" "InterruptForceOnce" {
      tunnel: "InterruptForceNumber" -> [_ w172]
      frame False {
      }
      frame True {
        n71 = call <vilib>:"niFPGA Interrupt.vi"("Wait Until Cleared (F)"=FALSE, "IRQ Number (0)"=w172) -> ()  [unwired: 1 in]
      }
    }
  }
  n72 = while {
    tunnel: w8 -> [w174]
    stop <- FALSE stop-if-true
    n73 = flat-sequence {
      tunnel: w174 -> [w176]
      frame #0 {
        n74 = Wait on Occurrence(2:w176) -> ()  [unwired: 2 in, 1 out]
      }
      frame #1 {
        n75 = case shown="True" "Alarm_Enable" {
          frame False {
          }
          frame True {
            n76 = call <vilib>:"niFPGA Interrupt.vi"("IRQ Number (0)"=u8 28) -> ()  [unwired: 2 in]
          }
        }
      }
    }
  }
  n77 = while {
    stop <- FALSE stop-if-true
    n78 = flat-sequence {
      tunnel: [w185] -> w182
      tunnel: [w184] -> w181
      tunnel: [w183] -> w180
      tunnel: w182 -> [w188]
      tunnel: w181 -> [w187]
      tunnel: w180 -> [w186]
      frame #0 {
        n79 = xnode "FPGA I/O Node"() -> ("AccelerationX"=w183:i16, "AccelerationY"=w184:i16, "AccelerationZ"=w185:i16)  [unwired: 3 in, 3 out]
      }
      frame #1 {
        "AccelerationZ" <- w188
        "AccelerationY" <- w187
        "AccelerationX" <- w186
      }
    }
  }
  n80 = node-c288() -> (w14:T17)  [unwired: 1 in]
  n81 = node-c288() -> (w16:T17)  [unwired: 1 in]
  n82 = timed-loop {
    timing: w12 -> [_]
    timing-out: [_] -> w11
    shift-right: [w190] -> _
    shift-left: _ -> [w189]
    stop <- _ stop-if-true
    w191 = u32 4000000 ("y")
    # "100 ms"
    n83 = Less?(x=w189, y=w191) -> (x < y?=w196:bool)
    "PWM_Enabled" <- w196
    n84 = Increment(x=w189) -> (x+1=w195:u32)
    n85 = Select(t=w195, s=w196, f=w191) -> (s? t:f=w194:u32)
    n86 = Select(t=u32 0, s="PWM_FeedWatchdog", f=w194) -> (s? t:f=w190:u32)
  }
  n87 = timed-loop {
    timing: w10 -> [_]
    timing-out: [_] -> w9
    stop <- _ stop-if-true
    n88 = call "DigitalOutputs.vi"("SPI_DIOEnable"="SPI_DIOEnable", "Digital_Outputs"="Digital_Outputs", "Digital_Output_Directions"="Digital_Output_Directions") -> ()
  }
  n89 = timed-loop {
    timing: w14 -> [_]
    timing-out: [_] -> w13
    stop <- _ stop-if-true
    n90 = xnode "FPGA I/O Node"() -> ("User Button"=→"User_Button":bool)  [unwired: 1 in, 1 out]
    n91 = xnode "FPGA I/O Node"("Radio LED Green"="Radio_LED_Green", "Radio LED Red"="Radio_LED_Red", "Comm LED Green"="Comm_LED_Green", "Comm LED Red"="Comm_LED_Red", "Mode LED Green"="Mode_LED_Green", "Mode LED Red"="Mode_LED_Red") -> ()  [unwired: 6 in, 6 out]
  }
  n92 = timed-loop {
    timing: w16 -> [_]
    timing-out: [_] -> w15
    stop <- _ stop-if-true
    n93 = Number To Boolean Array(number="Relay0") -> (Boolean array=w231:bool[])
    n94 = Number To Boolean Array(number="Relay1") -> (Boolean array=w226:bool[])
    n95 = Number To Boolean Array(number="Relay2") -> (Boolean array=w225:bool[])
    n96 = Number To Boolean Array(number="Relay3") -> (Boolean array=w222:bool[])
    n97 = Array To Cluster(array=w231) -> (cluster=w230:T21)
    n98 = Array To Cluster(array=w226) -> (cluster=w227:T21)
    n99 = Array To Cluster(array=w225) -> (cluster=w224:T21)
    n100 = Array To Cluster(array=w222) -> (cluster=w223:T21)
    n101 = Unbundle(w230) -> ("Boolean array[0]"=w229:bool, "Boolean array[1]"=w228:bool)
    n102 = Unbundle(w227) -> ("Boolean array[0]"=w213:bool, "Boolean array[1]"=w214:bool)
    n103 = Unbundle(w224) -> ("Boolean array[0]"=w215:bool, "Boolean array[1]"=w216:bool)
    n104 = Unbundle(w223) -> ("Boolean array[0]"=w218:bool, "Boolean array[1]"=w217:bool)
    n105 = xnode "FPGA I/O Node"("RelayFwd0"=w229, "RelayRev0"=w228, "RelayFwd1"=w213, "RelayRev1"=w214, "RelayFwd2"=w215, "RelayRev2"=w216, "RelayFwd3"=w218, "RelayRev3"=w217) -> ()  [unwired: 8 in, 8 out]
  }
  n106 = node-c288(w11) -> ()
  n107 = node-c288(w9) -> ()
  n108 = node-c288(w15) -> ()
  n109 = node-c288(w13) -> ()
  n110 = call "InterruptOccuranceGenerator.vi"() -> ("Occurances"=w5:T22)
  n111 = call "InterruptIRQs.vi"("Occurances"=w5) -> ()
  n112 = node-c288(w17) -> ()
  n113 = node-c288() -> (w7:T17)  [unwired: 1 in]
  n114 = timed-loop {
    timing: w7 -> [_]
    timing-out: [_] -> w6
    tunnel: w5 -> [w340]
    stop <- _ stop-if-true
    n115 = local read "Timing_Lower"() -> (w339:u32)
    n116 = flat-sequence {
      tunnel: [w349] -> w345
      tunnel: [w347] -> _
      tunnel: [w347] -> _
      frame #0 {
        # "Digital Inputs"
        n117 = call "DigitalInputs.vi"() -> ("NumInputs"=→"Num_Digital_Inputs":u8, "Outputs"=w349:bool[])
        n118 = Boolean Array To Number(Boolean array=w349) -> (number=w347:u32)
        "Digital_Inputs" <- w347
      }
    }
    n119 = local read "AnalogInputs"() -> (w338:u16[])
    n120 = feedback #1() -> (w346:T1[])  [unwired: 1 in]
    n121 = call "DutyCycles.vi"("AnalogTriggers"=w346, "DigitalInputs"=w345, "Sources"="DutyCycle_Sources") -> ("Frequencies"=w337:T23, "Outputs"=w328:T24)
    n122 = Unbundle(w337) -> ("DutyCycle0_Frequency"=→"DutyCycle0_Frequency":fxp<+,11,11>, "DutyCycle1_Frequency"=→"DutyCycle1_Frequency":fxp<+,11,11>, "DutyCycle2_Frequency"=→"DutyCycle2_Frequency":fxp<+,11,11>, "DutyCycle3_Frequency"=→"DutyCycle3_Frequency":fxp<+,11,11>, "DutyCycle4_Frequency"=→"DutyCycle4_Frequency":fxp<+,11,11>, "DutyCycle5_Frequency"=→"DutyCycle5_Frequency":fxp<+,11,11>, "DutyCycle6_Frequency"=→"DutyCycle6_Frequency":fxp<+,11,11>, "DutyCycle7_Frequency"=→"DutyCycle7_Frequency":fxp<+,11,11>)
    n123 = call "AnalogTriggers.vi"("Limits"="AnalogTrigger_Limits", "Sources"="AnalogTrigger_Sources", "DutyCycles"=w328, "AnalogInputs"=w338) -> ("Outputs"=w259:T25)
    n124 = Cluster To Array(cluster=w259) -> (array=w344:T1[])
    n125 = feedback-in #1(w344) -> ()
    n126 = Unbundle(w328) -> ("DutyCycle0_Output"=→"DutyCycle0_Output":fxp<+,31,31>, "DutyCycle1_Output"=→"DutyCycle1_Output":fxp<+,31,31>, "DutyCycle2_Output"=→"DutyCycle2_Output":fxp<+,31,31>, "DutyCycle3_Output"=→"DutyCycle3_Output":fxp<+,31,31>, "DutyCycle4_Output"=→"DutyCycle4_Output":fxp<+,31,31>, "DutyCycle5_Output"=→"DutyCycle5_Output":fxp<+,31,31>, "DutyCycle6_Output"=→"DutyCycle6_Output":fxp<+,31,31>, "DutyCycle7_Output"=→"DutyCycle7_Output":fxp<+,31,31>)
    n127 = Unbundle(w259) -> ("AT0_Output"=→"AT0_Output":T1, "AT1_Output"=→"AT1_Output":T1, "AT2_Output"=→"AT2_Output":T1, "AT3_Output"=→"AT3_Output":T1, "AT4_Output"=→"AT4_Output":T1, "AT5_Output"=→"AT5_Output":T1, "AT6_Output"=→"AT6_Output":T1, "AT7_Output"=→"AT7_Output":T1)
    n128 = Bundle("Counter0_Reset"="Counter0_Reset", "Counter1_Reset"="Counter1_Reset", "Counter2_Reset"="Counter2_Reset", "Counter3_Reset"="Counter3_Reset", "Counter4_Reset"="Counter4_Reset", "Counter5_Reset"="Counter5_Reset", "Counter6_Reset"="Counter6_Reset", "Counter7_Reset"="Counter7_Reset") -> (w297:T26)  [unwired: 1 in]
    n129 = call "InterruptsGroup.vi"("AnalogTriggers"=w344, "DigitalInputs"=w345, "SystemTime"=w339, "Configs"="Interrupts_Configs", "Occurances"=w340) -> ("Timestamps"=w260:T27)
    n130 = Unbundle(w260) -> ("Interrupt0_RisingTimestamp"=→"Interrupt0_RisingTimestamp":u32, "Interrupt0_FallingTimestamp"=→"Interrupt0_FallingTimestamp":u32, "Interrupt1_RisingTimestamp"=→"Interrupt1_RisingTimestamp":u32, "Interrupt1_FallingTimestamp"=→"Interrupt1_FallingTimestamp":u32, "Interrupt2_RisingTimestamp"=→"Interrupt2_RisingTimestamp":u32, "Interrupt2_FallingTimestamp"=→"Interrupt2_FallingTimestamp":u32, "Interrupt3_RisingTimestamp"=→"Interrupt3_RisingTimestamp":u32, "Interrupt3_FallingTimestamp"=→"Interrupt3_FallingTimestamp":u32, "Interrupt4_RisingTimestamp"=→"Interrupt4_RisingTimestamp":u32, "Interrupt4_FallingTimestamp"=→"Interrupt4_FallingTimestamp":u32, "Interrupt5_RisingTimestamp"=→"Interrupt5_RisingTimestamp":u32, "Interrupt5_FallingTimestamp"=→"Interrupt5_FallingTimestamp":u32, "Interrupt6_RisingTimestamp"=→"Interrupt6_RisingTimestamp":u32, "Interrupt6_FallingTimestamp"=→"Interrupt6_FallingTimestamp":u32, "Interrupt7_RisingTimestamp"=→"Interrupt7_RisingTimestamp":u32, "Interrupt7_FallingTimestamp"=→"Interrupt7_FallingTimestamp":u32)
    n131 = call "Counters.vi"("DigitalInputs"=w345, "AnalogTriggers"=w344, "Counter_TimerConfigs"="Counter_TimerConfigs", "Configs"="Counter_Configs", "Resets"=w297) -> ("Counter_Outputs"=w295:T28, "Counter_TimerOutputs"=w296:T29)
    n132 = Bundle("Encoder0_Reset"="Encoder0_Reset", "Encoder1_Reset"="Encoder1_Reset", "Encoder2_Reset"="Encoder2_Reset", "Encoder3_Reset"="Encoder3_Reset", "Encoder4_Reset"="Encoder4_Reset", "Encoder5_Reset"="Encoder5_Reset", "Encoder6_Reset"="Encoder6_Reset", "Encoder7_Reset"="Encoder7_Reset") -> (w306:T30)  [unwired: 1 in]
    n133 = call "Encoders.vi"("DigitalInputs"=w345, "AnalogTriggers"=w344, "Resets"=w306, "Configs"="Encoder_Configs", "TimerConfigs"="Encoder_TimerConfigs") -> ("Outputs"=w294:T31, "TimerOutputs"=w293:T32)
    n134 = Unbundle(w295) -> ("Counter0_Output"=→"Counter0_Output":T3, "Counter1_Output"=→"Counter1_Output":T3, "Counter2_Output"=→"Counter2_Output":T3, "Counter3_Output"=→"Counter3_Output":T3, "Counter4_Output"=→"Counter4_Output":T3, "Counter5_Output"=→"Counter5_Output":T3, "Counter6_Output"=→"Counter6_Output":T3, "Counter7_Output"=→"Counter7_Output":T3)
    n135 = Unbundle(w296) -> ("Counter0_TimerOutput"=→"Counter0_TimerOutput":T2, "Counter1_TimerOutput"=→"Counter1_TimerOutput":T2, "Counter2_TimerOutput"=→"Counter2_TimerOutput":T2, "Counter3_TimerOutput"=→"Counter3_TimerOutput":T2, "Counter4_TimerOutput"=→"Counter4_TimerOutput":T2, "Counter5_TimerOutput"=→"Counter5_TimerOutput":T2, "Counter6_TimerOutput"=→"Counter6_TimerOutput":T2, "Counter7_TimerOutput"=→"Counter7_TimerOutput":T2)
    n136 = Unbundle(w294) -> ("Encoder0_Output"=→"Encoder0_Output":T4, "Encoder1_Output"=→"Encoder1_Output":T4, "Encoder2_Output"=→"Encoder2_Output":T4, "Encoder3_Output"=→"Encoder3_Output":T4, "Encoder4_Output"=→"Encoder4_Output":T4, "Encoder5_Output"=→"Encoder5_Output":T4, "Encoder6_Output"=→"Encoder6_Output":T4, "Encoder7_Output"=→"Encoder7_Output":T4)
    n137 = Unbundle(w293) -> ("Encoder0_TimerOutput"=→"Encoder0_TimerOutput":T2, "Encoder1_TimerOutput"=→"Encoder1_TimerOutput":T2, "Encoder2_TimerOutput"=→"Encoder2_TimerOutput":T2, "Encoder3_TimerOutput"=→"Encoder3_TimerOutput":T2, "Encoder4_TimerOutput"=→"Encoder4_TimerOutput":T2, "Encoder5_TimerOutput"=→"Encoder5_TimerOutput":T2, "Encoder6_TimerOutput"=→"Encoder6_TimerOutput":T2, "Encoder7_TimerOutput"=→"Encoder7_TimerOutput":T2)
  }
  n138 = node-c288(w19) -> ()
  n139 = node-c288() -> (w4:T17)  [unwired: 1 in]
  n140 = timed-loop {
    timing: w4 -> [_]
    timing-out: [_] -> w3
    stop <- _ stop-if-true
  }
  n141 = node-c288(w1) -> ()
  n142 = node-c288(w3) -> ()
  n143 = node-c288(w6) -> ()
